vi "Assign GPIO.vi"(7 "SCK":T1=-1, 8 "error in (no error)":errorcluster, 9 "RX":T1=-1, 10 "TX":T1=-1, 11 "SPI in":refnum<class "SPI.lvclass">) -> (0 "error out":errorcluster, 3 "SPI out":refnum<class "SPI.lvclass">)   [LabVIEW 2024, in "CTI.lvlib" / "SPI.lvclass"]
uses:
  SPI.lvclass
  GPIO Number.ctl
  SPI.lvclass/SPI.ctl
  CTI.lvlib
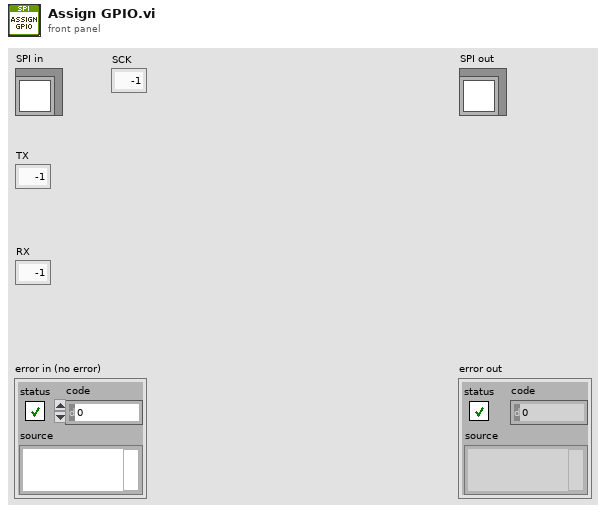
[diagram p1: front panel]
types:
  T1 = typedef "CTI.lvlib/GPIO Number.ctl" = i8
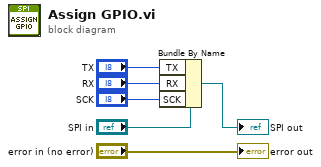
[diagram p0: block diagram]
diagram:
  n1 = Bundle By Name(cluster="SPI in", "TX"="TX", "RX"="RX", "SCK"="SCK") -> (→"SPI out":refnum<class "SPI.lvclass">)
  "error out" <- "error in (no error)"
